vi "Multi_channel_Voltage_Continuous_Output.vi"() -> ()   [LabVIEW 2018]
doc: "This example demonstrates how to continuously re-generate analog output data from a buffer in your computer's memory.\n\nRefer to your device documentation for pinouts and hardware capabilities."
uses:
  <vilib>/Utility/error.llb/DialogType.ctl
  <vilib>/DAQmx/write.llb/DAQmx Write (Analog 1D Wfm NChan NSamp).vi
  <vilib>/DAQmx/create/channels.llb/DAQmx Create Channel (AO-Voltage-Basic).vi
  <vilib>/DAQmx/configure/timing.llb/DAQmx Timing (Sample Clock).vi
  <vilib>/DAQmx/configure/trigger.llb/DAQmx Start Trigger (Digital Edge).vi
  <vilib>/DAQmx/configure/trigger.llb/DAQmx Start Trigger (Time).vi
  <vilib>/DAQmx/configure/trigger.llb/DAQmx Start Trigger (Analog Edge).vi
  <vilib>/DAQmx/miscellaneous.llb/DAQmx Fill In Error Info.vi
  <resource>/objmgr/daqmx.rc
  <vilib>/measure/NI_MABase.lvlib
panel:
  in  "Trigger Type":T1(tab)
  in  "Digital Start Trigger Edge":i32(ring)=10280 caption="Edge" items=["Rising"=10280, "Falling"=10171]
  in  "Digital Start Trigger Source":tag="/Dev1/PFI0" caption="Source"
  in  "Digital Pause Trigger Pause When":i32(ring)=10192 caption="Pause When" items=["High"=10192, "Low"=10214]
  in  "Digital Pause Trigger Source":tag="/Dev1/PFI0" caption="Source"
  in  "Analog Start Trigger Level":dbl caption="Level" format="%0.2f"
  in  "Analog Start Trigger Hysteresis":dbl caption="Hysteresis" format="%.2f"
  in  "Analog Start Trigger Slope":i32(ring)=10280 caption="Slope" items=["Rising"=10280, "Falling"=10171]
  in  "Analog Start Trigger Source":string="APFI0" caption="Source"
  in  "Analog Pause Trigger Source":string="APFI0" caption="Source"
  in  "Analog Pause Trigger Pause When":i32(ring)=10093 caption="Pause When" items=["Above Level"=10093, "Below Level"=10107]
  in  "Analog Pause Trigger Level":dbl caption="Level" format="%.2f"
  in  "When":timestamp
  in  "Select Time\nManually":bool
  in  "Output Array":T2(array[cluster])=[{"Waveform Type"=0, "Amplitude"=1.0, "Frequency"=10.0}] {"Frequency" format="%0.2p"; "Amplitude" format="%0.2p"; "Waveform Type" items=["Sine Wave", "Triangle Wave", "Square Wave", "Sawtooth Wave"]}
  in  "Number of Samples":i32=1000
  in  "Stop":bool
  out "Waveform Graph":waveform(dbl)[](graph)=[{"t0"=timestamp(0 s since 1904-01-01), "dt"=0.001, "Y"=[]}]
  in  "Sample Rate":dbl=1000.0
  in  "Sample Clock Source":tag="OnboardClock"
  in  "Max Voltage":dbl=5.0
  in  "Min Voltage":dbl=-5.0
  in  "Physical Channel(s)":tag="Dev1/ao0"
  out "Actual Sample Rate":dbl=1000.0 format="%0.2f"
  # "Channel Settings"
  # "Output"
  # "Timing and\nBuffer Settings"
  # "Waveform Settings"
  # "Trigger Settings"
  # "The number of elements in the waveform array must equal the number of channels in the task."
  # "To enable triggers, select a tab above, and configure the settings.\n\nNot all hardware supports all trigger types. Refer to your device documentation for more information."
  # "This trigger type is not supported in output tasks. \n\nRefer to your device documentation for more information on which triggers are supported."
  # "This trigger type is not supported in output tasks. \n\nRefer to your device documentation for more information on which triggers are supported."
  # "If time is not manually set, task will begin after 10 seconds"
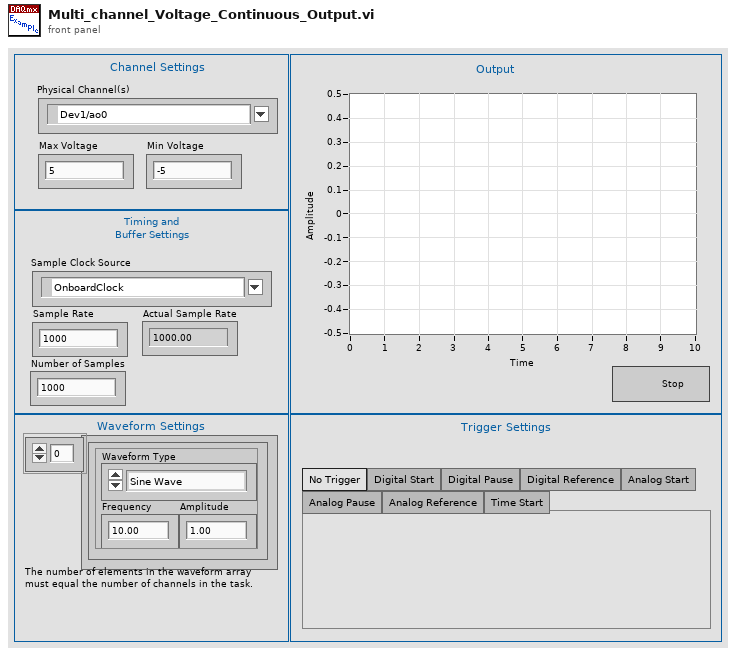
[diagram p1: front panel]
types:
  T1 = enum32{"No Trigger", "Digital Start", "Digital Pause", "Digital Reference", "Analog Start", "Analog Pause", "Analog Reference", "Time Start"}
  T2 = cluster{"Waveform Type":u16, "Amplitude":dbl, "Frequency":dbl}[]
  T3 = typedef "DialogType.ctl" = u16
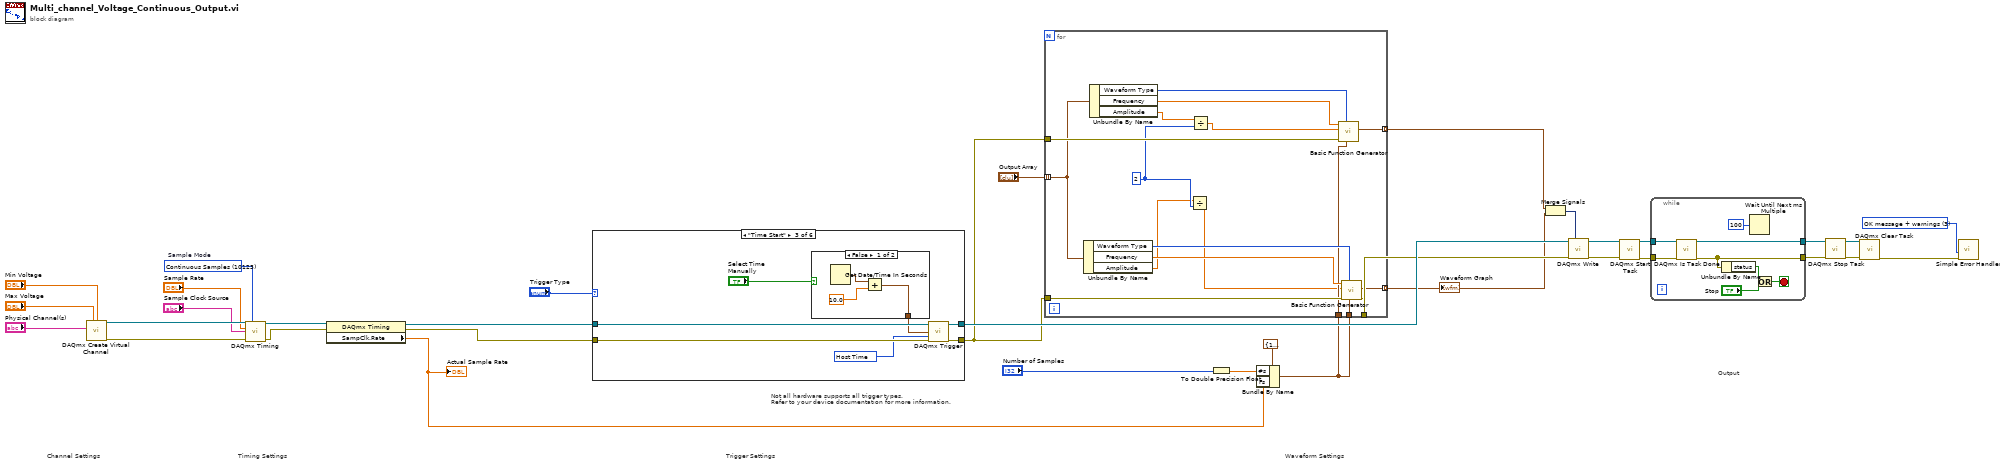
[diagram p0: block diagram]
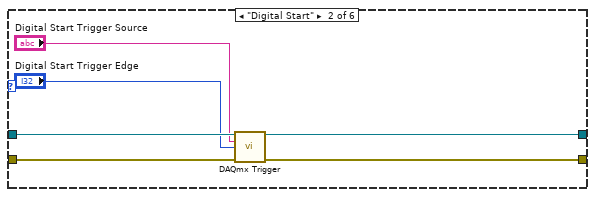
[diagram p3: hidden frame]
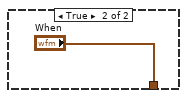
[diagram p4: hidden frame]
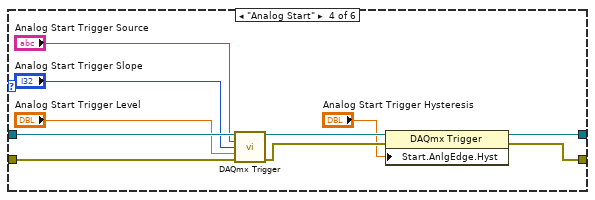
[diagram p5: hidden frame]
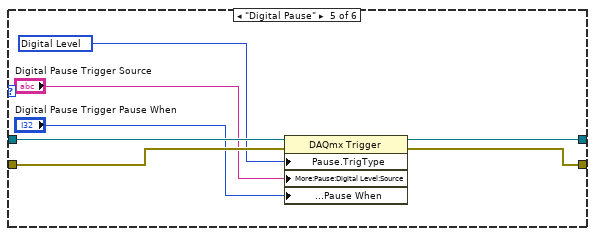
[diagram p6: hidden frame]
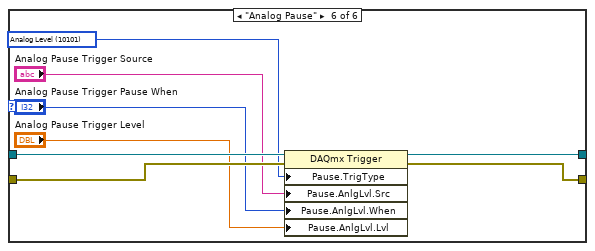
[diagram p7: hidden frame]
diagram:
  w12 = T3 3 items=["no dialog", "OK message", "continue or stop message", "OK message + warnings", "continue/stop + warnings"] ("type of dialog (OK msg:1)")
  w33 = 10123 items=["Finite Samples"=10178, "Continuous Samples"=10123, "Hardware Timed Single Point"=12522]  # Sample Mode
  # "Trigger Settings"
  # "Not all hardware supports all trigger types.\nRefer to your device documentation for more information."
  # "Output"
  # "Waveform Settings"
  # "Timing Settings"
  # "Channel Settings"
  n1 = call-poly <vilib>:"DAQmx Create Virtual Channel.vi"("maximum value"="Max Voltage", "minimum value"="Min Voltage", "physical channels"="Physical Channel(s)") -> ("task out"=w31:refnum<k21>, "error out"=w32:errorcluster)  [unwired: 11 in]
  n2 = call-poly <vilib>:"DAQmx Timing.vi"("task/channels in"=w31, "sample mode"=w33, "rate"="Sample Rate", "source"="Sample Clock Source", "error in"=w32) -> ("task out"=w35:refnum<k21>, "error out"=w34:errorcluster)  [unwired: 9 in]
  n3 = property class="DAQmx Timing"(reference=w35, error in=w34) -> (reference out=w10:refnum<k21>, error out=w9:errorcluster, "SampClk.Rate"=w7:dbl)
  "Actual Sample Rate" <- w7
  n4 = case shown="\"Time Start\"" "Trigger Type" {
    tunnel: w10 -> [w37 w43 w50 w64 w71 w79]
    tunnel: w9 -> [w36 w42 w49 w63 w68 w76]
    tunnel: [w37 w41 w48 w61 w70 w78] -> w8
    tunnel: [w36 w40 w47 w60 w69 w77] -> w3
    frame "No Trigger", Default {
    }
    frame "Digital Start" {
      n5 = call-poly <vilib>:"DAQmx Trigger.vi"("task/channels in"=w43, "source"="Digital Start Trigger Source", "edge"="Digital Start Trigger Edge", "error in"=w42) -> ("task out"=w41:refnum<k21>, "error out"=w40:errorcluster)  [unwired: 10 in]
    }
    frame "Time Start" {
      w46 = 16126 items=["Host Time"=16126, "I/O Device Time"=16127] ("timescale")
      n6 = case shown="False" "Select Time\nManually" {
        tunnel: [w52 "When"] -> w44
        frame False {
          n7 = Get Date/Time In Seconds() -> (seconds since 1Jan1904=w53:timestamp)
          n8 = Add(x=w53, y=10.0) -> (x+y=w52:timestamp)
        }
        frame True {
        }
      }
      n9 = call-poly <vilib>:"DAQmx Trigger.vi"("task/channels in"=w50, "when"=w44, "timescale"=w46, "error in"=w49) -> ("task out"=w48:refnum<k21>, "error out"=w47:errorcluster)  [unwired: 10 in]
    }
    frame "Analog Start" {
      n10 = call-poly <vilib>:"DAQmx Trigger.vi"("task/channels in"=w64, "source"="Analog Start Trigger Source", "slope"="Analog Start Trigger Slope", "level"="Analog Start Trigger Level", "error in"=w63) -> ("task out"=w59:refnum<k21>, "error out"=w58:errorcluster)  [unwired: 9 in]
      n11 = property class="DAQmx Trigger"(reference=w59, error in=w58, "Start.AnlgEdge.Hyst"="Analog Start Trigger Hysteresis") -> (reference out=w61:refnum<k21>, error out=w60:errorcluster)
    }
    frame "Digital Pause" {
      w67 = 10152 items=["Analog Level"=10101, "Analog Window"=10103, "Digital Level"=10152, "Digital Pattern"=10398, "None"=10230] ("Pause.TrigType")
      n12 = property class="DAQmx Trigger"(reference=w71, error in=w68, "Pause.TrigType"=w67, "More:Pause:Digital Level:Source"="Digital Pause Trigger Source", "More:Pause:Digital Level:Pause When"="Digital Pause Trigger Pause When") -> (reference out=w70:refnum<k21>, error out=w69:errorcluster)
    }
    frame "Analog Pause" {
      w75 = 10101 items=["Analog Level"=10101, "Analog Window"=10103, "Digital Level"=10152, "Digital Pattern"=10398, "None"=10230] ("Pause.TrigType")
      n13 = property class="DAQmx Trigger"(reference=w79, error in=w76, "Pause.TrigType"=w75, "Pause.AnlgLvl.Src"="Analog Pause Trigger Source", "Pause.AnlgLvl.When"="Analog Pause Trigger Pause When", "Pause.AnlgLvl.Lvl"="Analog Pause Trigger Level") -> (reference out=w78:refnum<k21>, error out=w77:errorcluster)
    }
  }
  n14 = To Double Precision Float(number="Number of Samples") -> (double precision float=w18:dbl)
  n15 = Bundle By Name(cluster=cluster{"Fs":dbl, "#s":dbl} {"Fs"=1000.0, "#s"=1000.0} ("sampling info"), "#s"=w18, "Fs"=w7) -> (w4:cluster{"Fs":dbl, "#s":dbl})
  n16 = for {
    tunnel: w3 -> [w96]
    tunnel: w4 -> [w95]
    tunnel: [w94] -> w5
    tunnel: "Output Array" -> [w85] mode=indexing
    tunnel: [w91] -> w2 mode=indexing
    tunnel: w3 -> [w88]
    tunnel: [w87] -> w1 mode=indexing
    tunnel: w4 -> [w86]
    w82 = 2
    n17 = Unbundle By Name(w85) -> ("Waveform Type"=w93:u16, "Frequency"=w92:dbl, "Amplitude"=w81:dbl)
    n18 = Unbundle By Name(w85) -> ("Waveform Type"=w89:u16, "Frequency"=w90:dbl, "Amplitude"=w84:dbl)
    n19 = Divide(x=w81, y=w82) -> (x/y=w80:dbl)
    n20 = Divide(x=w84, y=w82) -> (x/y=w83:dbl)
    n21 = call <vilib>:"Basic Function Generator.vi"("sampling info"=w86, "signal type"=w89, "error in (no error)"=w88, "amplitude"=w83, "frequency"=w90) -> ("signal out"=w87:waveform(dbl))  [unwired: 4 in, 2 out]
    n22 = call <vilib>:"Basic Function Generator.vi"("sampling info"=w95, "signal type"=w93, "error in (no error)"=w96, "amplitude"=w80, "frequency"=w92) -> ("error out"=w94:errorcluster, "signal out"=w91:waveform(dbl))  [unwired: 4 in, 1 out]
  }
  "Waveform Graph" <- w2
  n23 = Merge Signals(w1, w2) -> (w6:dynamicdata)
  n24 = call-poly <vilib>:"DAQmx Write.vi"("task/channels in"=w8, "data"=w6, "error in"=w5) -> ("task out"=w21:refnum<k21>, "error out"=w20:errorcluster)  [unwired: 10 in, 1 out]
  n25 = call <vilib>:"DAQmx Start Task.vi"("task/channels in"=w21, "error in"=w20) -> ("task out"=w30:refnum<k21>, "error out"=w29:errorcluster)  [unwired: 12 in]
  n26 = while {
    tunnel: w30 -> [w104]
    tunnel: w29 -> [w103]
    tunnel: [w100] -> w13
    tunnel: [w101] -> w14
    stop <- w102 stop-if-true
    n27 = call <vilib>:"DAQmx Is Task Done.vi"("task/channels in"=w104, "error in"=w103) -> ("task out"=w101:refnum<k21>, "error out"=w100:errorcluster)  [unwired: 11 in, 1 out]
    n28 = Unbundle By Name(w100) -> ("status"=w99:bool)
    n29 = Wait Until Next ms Multiple(millisecond multiple=u32 100) -> ()  [unwired: 1 out]
    n30 = Or(x=w99, y="Stop") -> (x .or. y?=w102:bool)
  }
  n31 = call <vilib>:"DAQmx Stop Task.vi"("task/channels in"=w14, "error in"=w13) -> ("task out"=w16:refnum<k21>, "error out"=w15:errorcluster)  [unwired: 12 in]
  n32 = call <vilib>:"DAQmx Clear Task.vi"("task in"=w16, "error in"=w15) -> ("error out"=w28:errorcluster)  [unwired: 13 in]
  n33 = call <vilib>:"Simple Error Handler.vi"("type of dialog (OK msg:1)"=w12, "error in (no error)"=w28) -> ()  [unwired: 3 in, 5 out]
